vi "RemoveFromMemory.vi"(8 "error in (no error)":errorcluster, 11 "ExcelFile in":refnum<class "PortableExcelFileManipulationOXML.lvclass">) -> (0 "error out":errorcluster)   [LabVIEW 2019, in "PortableExcelFileManipulationOXML.lvclass"]
doc: "Removes Excel File From Memory"
uses:
  PortableExcelFileManipulationOXML.lvclass
  PortableExcelFileManipulationOXML.lvclass/PortableExcelFileManipulationOXML.ctl
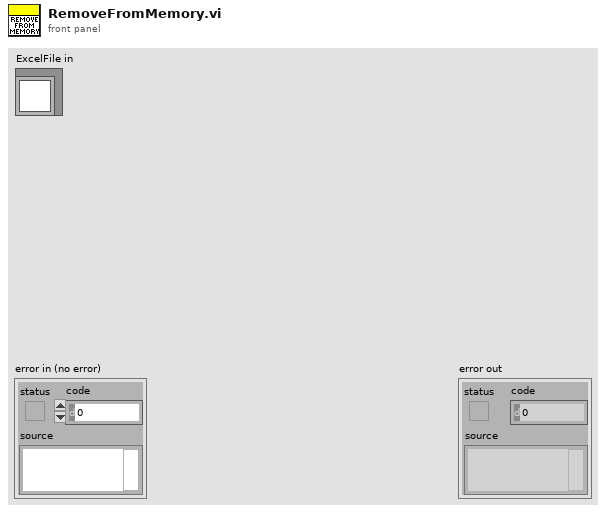
[diagram p1: front panel]
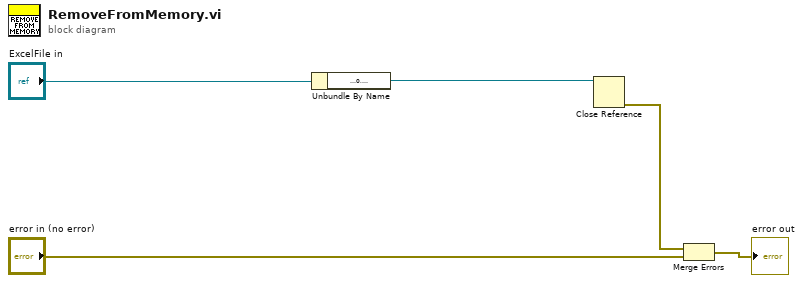
[diagram p0: block diagram]
diagram:
  n1 = Unbundle By Name("ExcelFile in") -> ("ExcelOpen"=w1:refnum<k24>)
  n2 = Close Reference(reference=w1) -> (error out=w4:errorcluster)  [unwired: 1 in]
  n3 = Merge Errors(w4, "error in (no error)") -> (→"error out":errorcluster)
